vi "AlliGator Plugin Target to Submenu.vi"(9 "Function Target Type":T1, 11 "Function Target":string) -> (3 "Menu Tag":string)   [LabVIEW 2021, in "AlliGator Python Plugins.lvlib"]
doc: "Convert Plugin Target to Menu Tag for insertion of the menu item.\n\nFor plugins associated with objects such as Source Image or Decay Graph, the insertion takes place at the bottom of contextual menu and thus an empty string is provided.\n\nFor plugins associated with data not exposed to the user (such as the Gate Series), the plugin menui is added to the main menu, and thus the tag of the submenu in which it will be inserted needs to be provided."
uses:
  AlliGator Python Plugins.lvlib
  AlliGator Python Plugin Target Type.ctl
panel:
  # "see the AlliGator License on the block diagram (Ctrl+E or Window:Show Block Diagram)"
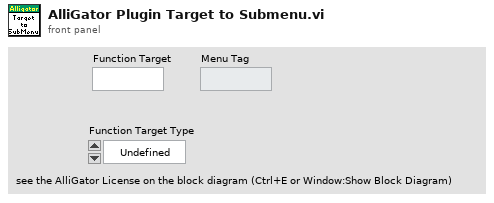
[diagram p1: front panel]
types:
  T1 = typedef "AlliGator Python Plugins.lvlib/AlliGator Python Plugin Target Type.ctl" = enum16{"Undefined", "Window Menu", "Object Menu"}
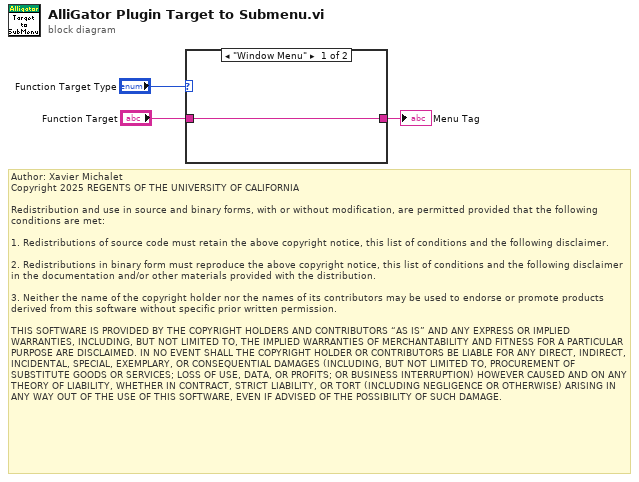
[diagram p0: block diagram]
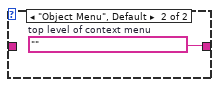
[diagram p2: hidden frame]
diagram:
  # "Author: Xavier Michalet\nCopyright 2025 REGENTS OF THE UNIVERSITY OF CALIFORNIA\n\nRedistribution and use in source and binary forms, with or without modification, are permitted provided that the following conditions are met:\n\n1. Redistributions of source code must retain the above copyright notice, this list of conditions and the following disclaimer.\n\n2. Redistributions in binary form must reproduce the above copyright notice, this list of conditions and the following disclaimer in the documentation and/or other materials provided with the distribution.\n\n3. Neither the name of the copyright holder nor the names of its contributors may be used to endorse or promote products derived from this software without specific prior written permission.\n\nTHIS SOFTWARE IS PROVIDED BY THE COPYRIGHT HOLDERS AND CONTRIBUTORS “AS IS” AND ANY EXPRESS OR IMPLIED WARRANTIES, INCLUDING, BUT NOT LIMITED TO, THE IMPLIED WARRANTIES OF MERCHANTABILITY AND FITNESS FOR A PARTICULAR PURPOSE ARE DISCLAIMED. IN NO EVENT SHALL THE COPYRIGHT HOLDER OR CONTRIBUTORS BE LIABLE FOR ANY DIRECT, INDIRECT, INCIDENTAL, SPECIAL, EXEMPLARY, OR CONSEQUENTIAL DAMAGES (INCLUDING, BUT NOT LIMITED TO, PROCUREMENT OF SUBSTITUTE GOODS OR SERVICES; LOSS OF USE, DATA, OR PROFITS; OR BUSINESS INTERRUPTION) HOWEVER CAUSED AND ON ANY THEORY OF LIABILITY, WHETHER IN CONTRACT, STRICT LIABILITY, OR TORT (INCLUDING NEGLIGENCE OR OTHERWISE) ARISING IN ANY WAY OUT OF THE USE OF THIS SOFTWARE, EVEN IF ADVISED OF THE POSSIBILITY OF SUCH DAMAGE."
  n1 = case shown="\"Window Menu\"" "Function Target Type" {
    tunnel: "Function Target" -> [w4 _]
    tunnel: [w4 w5] -> w1
    frame "Window Menu" {
    }
    frame "Object Menu", Default {
      w5 = ""  # top level of context menu
    }
  }
  "Menu Tag" <- w1
